vi "Help logger.vi"() -> ()   [LabVIEW 2018]
panel:
  out "EN help":string="S4ICS records events in files in order to help with maintenance and improvement. These records can be enabled or disabled in the LOG ENABLE control by inserting or removing the event level according to the following table:\n\n0: S4DMX program (running inside motors) errors.\n1: WPROT motor instructions (Immediate/Cyclic).\n2: Active motor instructions.\n3: TCP client commands.\n4: Status sent to TCP client.\n5. Position during movements.\nEXAMPLE:\nTo enable only the logging of level 1 and 3 events, leave LOG ENABLE = 13.\n" caption="LOG ENABLE"
  out "PT help":string="O S4ICS registra em arquivos eventos que podem auxiliar na manutenção e no seu aprimoramento. Esses registros podem ser habiitados ou desabilitados no controle LOG ENABLE inserindo ou removendo o nível do evento de acordo com a seguinte tabela:\n0: Erros no programa S4DMX (rodando no motor).\n1: Instruções do motor WPROT (Immediate/Cyclic).\n2: Instruções dos motores ativos.\n3: Comandos de cliente TCP.\n4: Resposta enviada a cliente TCP.\n5. Posição durante movimentos.\nEXEMPLO:\nPara habilitar apenas o registros dos eventos do nível 1 e 3, deixar LOG ENABLE = 13. \n" caption="HABILITAR LOG"
  in  "ok":bool
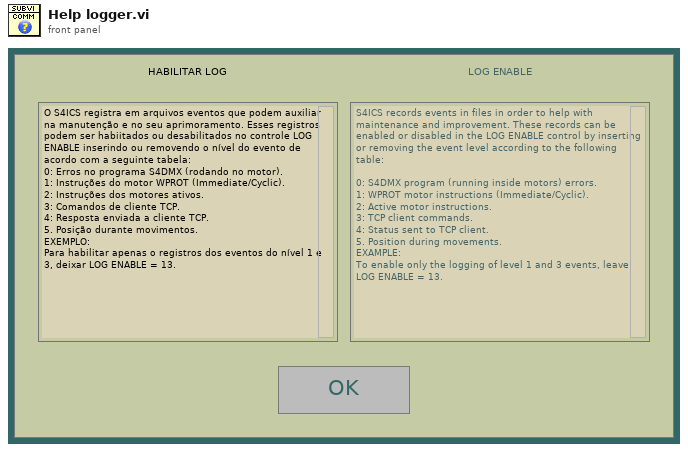
[diagram p1: front panel]
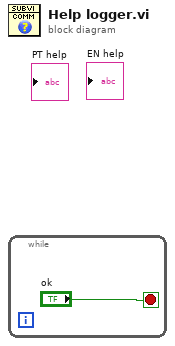
[diagram p0: block diagram]
diagram:
  n1 = while {
    stop <- "ok" stop-if-true
  }
